vi "for_condicional.vi"() -> ()   [LabVIEW 2020]
panel:
  out "Array 2":i32[](array[numeric])
  out "Array":dbl[](array[numeric])
  out "Thermometer":dbl(slide) scale=0.0..100.0
  out "Numeric":i32
  # "for"
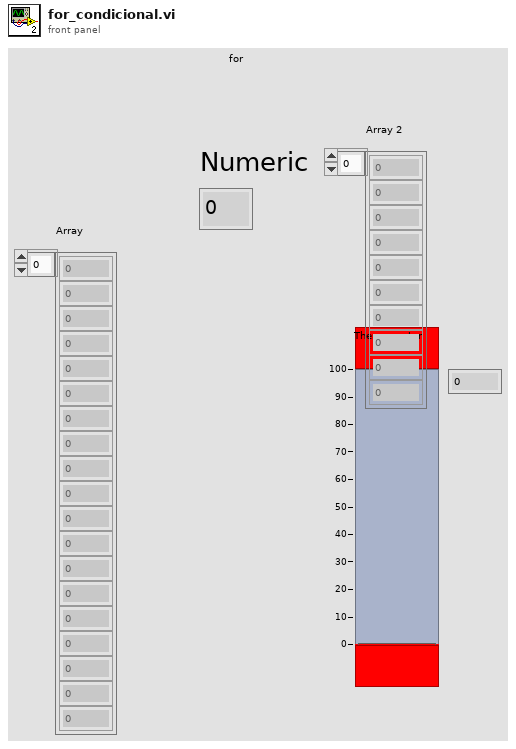
[diagram p1: front panel]
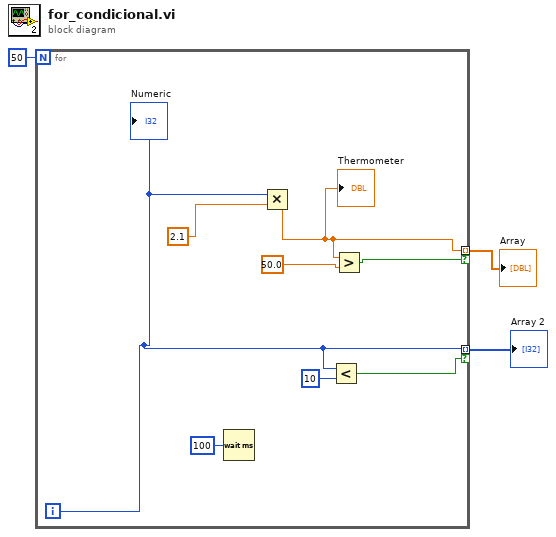
[diagram p0: block diagram]
diagram:
  n1 = for {
    N: 50 -> [_]
    tunnel: [w8] -> w2 mode=indexing if=w4
    tunnel: [w9] -> w1 mode=indexing if=w5
    i -> [w9]
    n2 = Wait (ms)(milliseconds to wait=u32 100) -> ()  [unwired: 1 out]
    n3 = Multiply(x=w9, y=2.1) -> (x*y=w8:dbl)
    "Thermometer" <- w8
    n4 = Less?(x=w9, y=10) -> (x < y?=w5:bool)
    n5 = Greater?(x=w8, y=50.0) -> (0:w4:bool)
    "Numeric" <- w9
  }
  "Array" <- w2
  "Array 2" <- w1
